vi "Get Data I16_32.vi"(8 "error in (no error)":errorcluster, 11 "Ni-Scope Digitizer in":refnum<class "Ni-Scope Digitizer.lvclass">) -> (0 "error out":errorcluster, 1 "I32 data out":i32[][](array[numeric]), 2 "I16 data out":i16[][](array[numeric]), 3 "Ni-Scope Digitizer out":refnum<class "Ni-Scope Digitizer.lvclass">, 4 "Finished":bool, 5 "Current read position":i32)   [LabVIEW 2016, in "Ni-Scope Digitizer.lvclass"]
uses:
  Ni-Scope Digitizer.lvclass
  C:/github/NHMFL_Core/Libraries/Instruments/Pulse Driver/Pulse Driver.lvclass
  Ni-Scope Digitizer.lvclass/Ni-Scope Digitizer.ctl
  Instruments/Pulse Driver/Pulse Driver.lvclass/Pulse Driver.ctl
  Instruments/Pulse Driver/Read Samples per channel.vi
  Instruments/Pulse Driver/Read Current read position.vi
  Instruments/Pulse Driver/Read Samples per read.vi
  Instruments/Pulse Driver/Read Binary sample width.vi
  Read Fetch Relative To.vi
  Write instrument handle.vi
  <instrlib>/niScope/Acquire/Fetch/niScope Multi Fetch Binary 16.vi
  <instrlib>/niScope/Acquire/Fetch/niScope Multi Fetch Binary 32.vi
panel:
  out "Horizontal:Reference Position":dbl
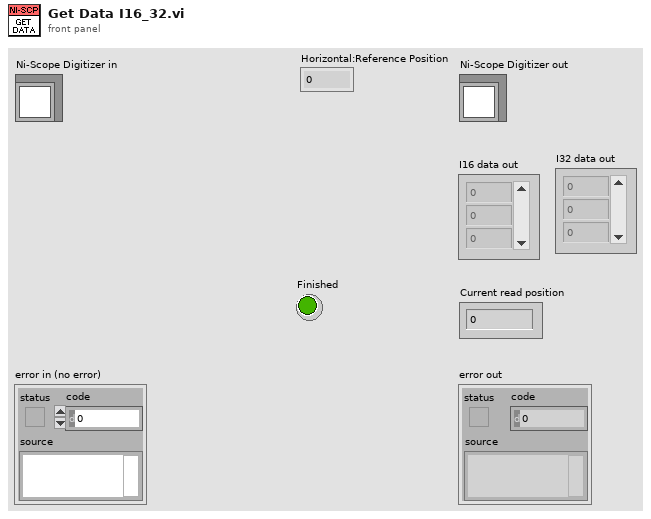
[diagram p1: front panel]
types:
  T1 = typedef "Pusle Driver Configuration.ctl" = cluster{"Pre-trigger duration":dbl, "Post-trigger duration":dbl, "Rate":dbl, "Ranges":dbl[], "Re-name channels":string[], "Active channels":string, "External clock":bool}
  T2 = cluster{"actualSamples":i32, "absoluteInitialX":dbl, "relativeInitialX":dbl, "xIncrement":dbl, "offset":dbl, "gain":dbl, "reserved1":dbl, "reserved2":dbl}[]
  T3 = cluster{"actualSamples":i32, "absoluteInitialX":dbl, "relativeInitialX":dbl, "xIncrement":dbl, "offset":dbl, "gain":dbl, "reserved1":dbl, "reserved2":dbl}
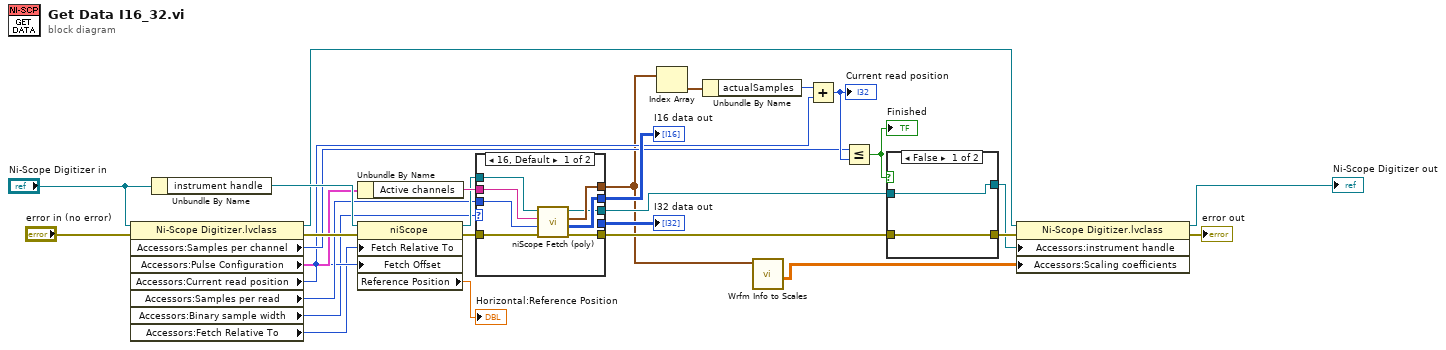
[diagram p0: block diagram]
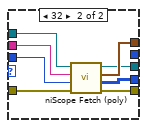
[diagram p2: hidden frame]
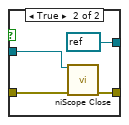
[diagram p3: hidden frame]
diagram:
  n1 = property class="Ni-Scope Digitizer.lvclass"(reference="Ni-Scope Digitizer in", error in="error in (no error)") -> (reference out=w5:refnum<class "Ni-Scope Digitizer.lvclass">, error out=w24:errorcluster, "Accessors:Samples per channel"=w15:i32, "Accessors:Pulse Configuration"=w14:T1, "Accessors:Current read position"=w11:i32, "Accessors:Samples per read"=w13:i32, "Accessors:Binary sample width"=w9:i32, "Accessors:Fetch Relative To"=w7:i32)
  n2 = Unbundle By Name("Ni-Scope Digitizer in") -> ("instrument handle"=w27:refnum<k15>)
  n3 = Unbundle By Name(w14) -> ("Active channels"=w29:string)
  n4 = property class="niScope"(reference=w27, error in=w24, "Fetch Relative To"=w7, "Fetch Offset"=w11) -> (reference out=w26:refnum<k15>, error out=w25:errorcluster, "Reference Position"=→"Horizontal:Reference Position":dbl)
  n5 = case shown="16, Default" w9 {
    tunnel: w29 -> [w37 w45]
    tunnel: w26 -> [w36 w44]
    tunnel: w25 -> [w35 w43]
    tunnel: [w34 w42] -> w22
    tunnel: [w33 _] -> w21
    tunnel: [w32 w41] -> w2
    tunnel: [w31 w40] -> w17
    tunnel: w13 -> [w30 w39]
    tunnel: [_ w38] -> w8
    frame 16, Default {
      n6 = call-poly <instrlib>:"niScope Fetch (poly).vi"("error in"=w35, "numSamples"=w30, "channels"=w37, "instrument handle"=w36) -> ("error out"=w34:errorcluster, "wfm"=w33:i16[][], "wfm info"=w32:T2, "instrument handle out"=w31:refnum<k15>)  [unwired: 4 in]
    }
    frame 32 {
      n7 = call-poly <instrlib>:"niScope Fetch (poly).vi"("error in"=w43, "numSamples"=w39, "channels"=w45, "instrument handle"=w44) -> ("error out"=w42:errorcluster, "wfm"=w38:i32[][], "wfm info"=w41:T2, "instrument handle out"=w40:refnum<k15>)  [unwired: 4 in]
    }
  }
  "I16 data out" <- w21
  "I32 data out" <- w8
  n8 = Index Array(array=w2) -> (element=w20:T3)  [unwired: 1 in]
  n9 = Unbundle By Name(w20) -> ("actualSamples"=w19:i32)
  n10 = call "Wrfm Info to Scales.vi"("wfm info"=w2) -> ("Scaling coefficients"=w1:dbl[][])  [unwired: 8 in, 2 out]
  n11 = Add(x=w19, y=w11) -> (x+y=w18:i32)
  "Current read position" <- w18
  n12 = Less Or Equal?(x=w15, y=w18) -> (x <= y?=w12:bool)
  "Finished" <- w12
  n13 = case shown="False" w12 {
    tunnel: [w47 w51] -> w16
    tunnel: w17 -> [w46 w50]
    tunnel: w22 -> [w47 w49]
    tunnel: [w46 refnum<k15> refnum ("instrument handle out")] -> w3
    frame False {
    }
    frame True {
      n14 = call <instrlib>:"niScope Close.vi"("instrument handle"=w50, "error in"=w49) -> ("error out"=w51:errorcluster)  [unwired: 13 out]
    }
  }
  n15 = property class="Ni-Scope Digitizer.lvclass"(reference=w5, error in=w16, "Accessors:instrument handle"=w3, "Accessors:Scaling coefficients"=w1) -> (reference out=→"Ni-Scope Digitizer out":refnum<class "Ni-Scope Digitizer.lvclass">, error out=→"error out":errorcluster)
